vi "initialise.vi"(8 "error in (no error)":errorcluster, 11 "GenericPlugin in":refnum<class "ClockMT120808DAQmxSimple.lvclass">) -> (0 "error out":errorcluster, 3 "GenericPlugin out":refnum<class "ClockMT120808DAQmxSimple.lvclass">)   [LabVIEW 2010, in "ClockMT120808DAQmxSimple.lvclass"]
doc: "The dynamic dispatch-version of this VI initalises the plug-in object by allocating and initalising any dynamic resources need."
uses:
  ClockMT120808DAQmxSimple.lvclass
  GenericClock/GenericClock/GenericClock.lvclass
  ClockMT120808DAQmxSimple.lvclass/ClockMT120808DAQmxSimple.ctl
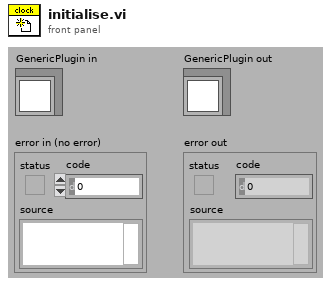
[diagram p1: front panel]
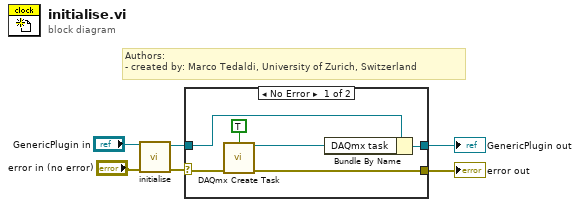
[diagram p0: block diagram]
diagram:
  # "Authors: \n- created by: Marco Tedaldi, University of Zurich, Switzerland"
  n1 = call-parent "initialise.vi"("error in (no error)"="error in (no error)", "GenericPlugin in"="GenericPlugin in") -> ("error out"=w4:errorcluster, "GenericPlugin out"=w3:refnum<class "ClockMT120808DAQmxSimple.lvclass">)  [unwired: 8 in]
  n2 = case shown="No Error" w4 {
    selector: w4 -> [w10 w14]
    tunnel: w3 -> [w8 w13]
    tunnel: [w9 w14] -> w2
    tunnel: [w7 w13] -> w1
    frame No Error {
      n3 = call <vilib>:"DAQmx Create Task.vi"("auto cleanup"=TRUE, "error in"=w10) -> ("task out"=w11:refnum<k21>, "error out"=w9:errorcluster)  [unwired: 12 in]
      n4 = Bundle By Name(cluster=w8, "DAQmx task"=w11) -> (w7:refnum<class "ClockMT120808DAQmxSimple.lvclass">)
    }
    frame Error {
    }
  }
  "error out" <- w2
  "GenericPlugin out" <- w1
